vi "Advance Balls SUBVI.vi"(11 "Numeric":dbl) -> ()   [LabVIEW 2011]
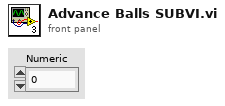
[diagram p1: front panel]
types:
  T1 = typedef "WPI_DigitalInputDevRef.ctl" = cluster{"DevStatus":errorcluster, "DIO Channel":T2, "Digital Module":T3}
  T2 = typedef "FPGA_DIOChannel.ctl" = enum8{"DIO 1", "DIO 2", "DIO 3", "DIO 4", "DIO 5", "DIO 6", "DIO 7", "DIO 8", "DIO 9", "DIO 10", "DIO 11", "DIO 12", "DIO 13", "DIO 14", "Invalid"}
  T3 = typedef "FPGA_TypedefDigitalModule.ctl" = enum16{"Digital Module 1", "Digital Module 2"}
  T4 = typedef "WPI_MotorControlDeviceRef.ctl" = cluster{"DeviceStatus":errorcluster, "Type":enum16{"PWM", "CAN"}, "PWM":cluster{"Digital Module":T3, "PWM Channel":T5, "DeadBand":T6}, "CAN":cluster{"Device Number":u8, "Control Mode":T7, "Semaphore":T8, "Max Vout":dbl}, "Invert":bool, "TransformRef":T9, "InvTransformRef":T9}
  T5 = typedef "FPGA_DIOPWMChannel.ctl" = enum8{"PWM 1", "PWM 2", "PWM 3", "PWM 4", "PWM 5", "PWM 6", "PWM 7", "PWM 8", "PWM 9", "PWM 10", "Invalid"}
  T6 = typedef "WPI_PWMDeadband.ctl" = cluster{"Name":string, "maxPositivePwm":i32, "minPositivePwm":i32, "centerPwm":i32, "maxNegativePwm":i32, "minNegativePwm":i32, "angularRange":u16}
  T7 = typedef "WPI_CANJaguar_ControlMode.ctl" = enum8{"Percent VBus", "Current", "Speed", "Position", "Voltage"}
  T8 = typedef "Semaphore RefNum" = refnum<k1>
  T9 = typedef "WPI_PWMTransform_ConPane.ctl" = refnum<vi>
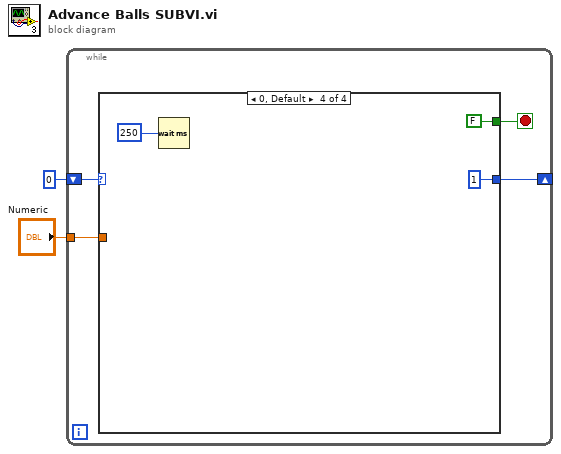
[diagram p0: block diagram]
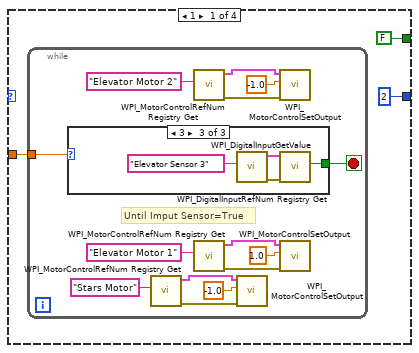
[diagram p2: hidden frame]
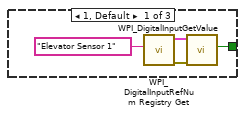
[diagram p3: hidden frame]
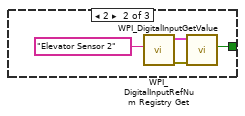
[diagram p4: hidden frame]
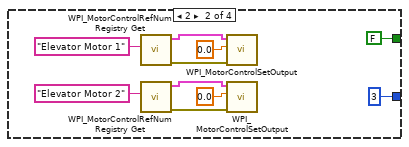
[diagram p5: hidden frame]
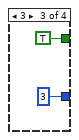
[diagram p6: hidden frame]
diagram:
  n1 = while {
    shift-right: [w5] -> _
    shift-left: 0 -> [w6]
    tunnel: "Numeric" -> [w3]
    stop <- w4 stop-if-true
    n2 = case shown="0, Default" w6 {
      tunnel: [2 3 3 1] -> w5
      tunnel: [FALSE FALSE TRUE FALSE] -> w4
      tunnel: w3 -> [w7 _ _ _]
      frame 1 {
        n3 = while {
          tunnel: w7 -> [w15]
          stop <- w14 stop-if-true
          # "Until Imput Sensor=True"
          n4 = case shown="3" w15 {
            tunnel: [w24 w28 w32] -> w14
            frame 1, Default {
              n5 = call <vilib>:"WPI_DigitalInputRefNum Registry Get.vi"("refnum name"="Elevator Sensor 1") -> ("error out"=w25:errorcluster, "DigitalInputDevRef"=w26:T1)  [unwired: 9 in]
              n6 = call <vilib>:"WPI_DigitalInputGetValue.vi"("error in (no error)"=w25, "DigitalInputDevRef"=w26) -> ("Value"=w24:bool)  [unwired: 7 in, 2 out]
            }
            frame 2 {
              n7 = call <vilib>:"WPI_DigitalInputRefNum Registry Get.vi"("refnum name"="Elevator Sensor 2") -> ("error out"=w29:errorcluster, "DigitalInputDevRef"=w30:T1)  [unwired: 9 in]
              n8 = call <vilib>:"WPI_DigitalInputGetValue.vi"("error in (no error)"=w29, "DigitalInputDevRef"=w30) -> ("Value"=w28:bool)  [unwired: 7 in, 2 out]
            }
            frame 3 {
              n9 = call <vilib>:"WPI_DigitalInputRefNum Registry Get.vi"("refnum name"="Elevator Sensor 3") -> ("error out"=w33:errorcluster, "DigitalInputDevRef"=w34:T1)  [unwired: 9 in]
              n10 = call <vilib>:"WPI_DigitalInputGetValue.vi"("error in (no error)"=w33, "DigitalInputDevRef"=w34) -> ("Value"=w32:bool)  [unwired: 7 in, 2 out]
            }
          }
          n11 = call <vilib>:"WPI_MotorControlRefNum Registry Get.vi"("refnum name"="Stars Motor") -> ("error out"=w10:errorcluster, "MotorControlDevRef"=w11:T4)  [unwired: 9 in]
          n12 = call <vilib>:"WPI_MotorControlRefNum Registry Get.vi"("refnum name"="Elevator Motor 2") -> ("error out"=w17:errorcluster, "MotorControlDevRef"=w18:T4)  [unwired: 9 in]
          n13 = call <vilib>:"WPI_MotorControlRefNum Registry Get.vi"("refnum name"="Elevator Motor 1") -> ("error out"=w20:errorcluster, "MotorControlDevRef"=w21:T4)  [unwired: 9 in]
          n14 = call <vilib>:"WPI_MotorControlSetOutput.vi"("error in (no error)"=w10, "Output"=-1.0, "MotorControlDevRef"=w11) -> ()  [unwired: 7 in, 2 out]
          n15 = call <vilib>:"WPI_MotorControlSetOutput.vi"("error in (no error)"=w17, "Output"=-1.0, "MotorControlDevRef"=w18) -> ()  [unwired: 7 in, 2 out]
          n16 = call <vilib>:"WPI_MotorControlSetOutput.vi"("error in (no error)"=w20, "Output"=1.0, "MotorControlDevRef"=w21) -> ()  [unwired: 7 in, 2 out]
        }
      }
      frame 2 {
        n17 = call <vilib>:"WPI_MotorControlRefNum Registry Get.vi"("refnum name"="Elevator Motor 1") -> ("error out"=w42:errorcluster, "MotorControlDevRef"=w43:T4)  [unwired: 9 in]
        n18 = call <vilib>:"WPI_MotorControlRefNum Registry Get.vi"("refnum name"="Elevator Motor 2") -> ("error out"=w39:errorcluster, "MotorControlDevRef"=w40:T4)  [unwired: 9 in]
        n19 = call <vilib>:"WPI_MotorControlSetOutput.vi"("error in (no error)"=w42, "Output"=0.0, "MotorControlDevRef"=w43) -> ()  [unwired: 7 in, 2 out]
        n20 = call <vilib>:"WPI_MotorControlSetOutput.vi"("error in (no error)"=w39, "Output"=0.0, "MotorControlDevRef"=w40) -> ()  [unwired: 7 in, 2 out]
      }
      frame 3 {
      }
      frame 0, Default {
        n21 = Wait (ms)(milliseconds to wait=250) -> ()  [unwired: 1 out]
      }
    }
  }
